vi "Convert Decimal Time to HMS.vi"(3 "Decimal Time":dbl=232.247881 format="%.6f") -> (1 "HMS Time":string="15:28:59.491")   [LabVIEW 2015]
panel:
  out "degrees left after hours removed":dbl=7.247881000000007
  out "Seconds":dbl=59.4914400000016 format="%.2f"
  out "Minutes":i16=28
  out "Hours":i16=15
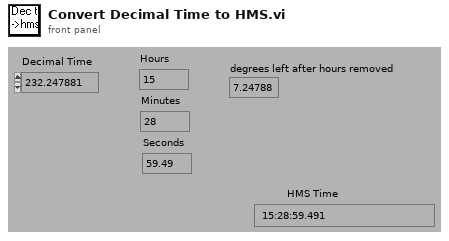
[diagram p1: front panel]
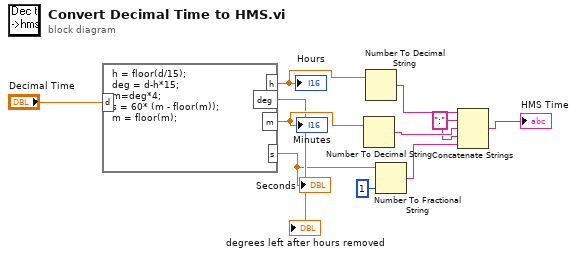
[diagram p0: block diagram]
diagram:
  w5 = ":" ("string")
  n1 = formula code="h = floor(d/15);\ndeg = d-h*15;\nm=deg*4;\ns = 60* (m - floor(m));\nm = floor(m);"("d"="Decimal Time") -> ("h"=w10:dbl, "m"=w8:dbl, "s"=w3:dbl, "deg"=→"degrees left after hours removed":dbl)
  "Hours" <- w10
  "Minutes" <- w8
  "Seconds" <- w3
  n2 = Number To Decimal String(number=w8) -> (decimal integer string=w6:string)  [unwired: 1 out]
  n3 = Number To Decimal String(number=w10) -> (decimal integer string=w7:string)  [unwired: 1 out]
  n4 = Number To Fractional String(number=w3, precision (6)=i16 1) -> (F-format string=w2:string)  [unwired: 2 out]
  n5 = Concatenate Strings(w7, w5, w6, w5, w2) -> (→"HMS Time":string)
